vi "IPS Parse Switch Heater.vi"(1 "Response":string) -> (0 "Switch Message":string)   [LabVIEW 2016, in "IPS-120.lvlib"]
uses:
  IPS-120.lvlib
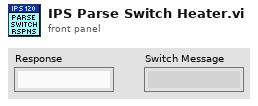
[diagram p1: front panel]
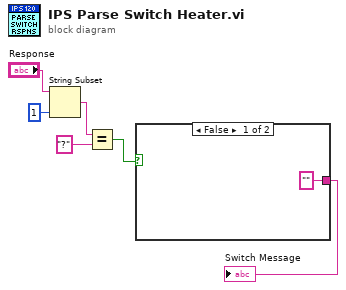
[diagram p0: block diagram]
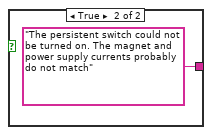
[diagram p2: hidden frame]
diagram:
  n1 = String Subset(string="Response", length (rest)=1 ("length (rest)")) -> (substring=w3:string)  [unwired: 1 in]
  n2 = Equal?(x=w3, y="?") -> (x = y?=w5:bool)
  n3 = case shown="False" w5 {
    tunnel: ["" ("Switch Message") "The persistent switch could not be turned on. The magnet and power supply currents probably do not match" ("Switch Message")] -> w6
    frame False {
    }
    frame True {
    }
  }
  "Switch Message" <- w6
